vi "Write Timeout.vi"(8 "error in (no error)":errorcluster, 10 "Timeout time(-1ms)":i32=-1, 11 "Interruptible Reply Core in":refnum<class "Interruptible Reply Core.lvclass">) -> (0 "error out":errorcluster, 3 "Interruptible Reply Core out":refnum<class "Interruptible Reply Core.lvclass">)   [LabVIEW 2020, in "Publisher.lvlib" / "Interruptible Reply Core.lvclass"]
doc: "Write the timeout time in ms."
uses:
  Interruptible Reply Core.lvclass
  Interruptible Reply Core.lvclass/Interruptible Reply Core.ctl
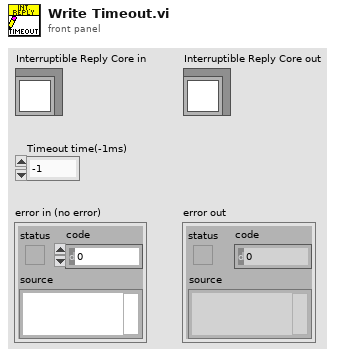
[diagram p1: front panel]
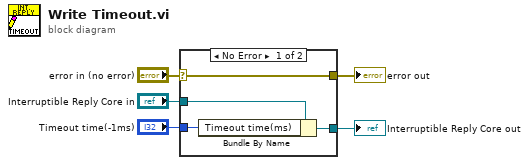
[diagram p0: block diagram]
diagram:
  n1 = case shown="No Error" "error in (no error)" {
    selector: "error in (no error)" -> [w9 w10]
    tunnel: [w9 w10] -> w4
    tunnel: [w7 w11] -> w2
    tunnel: "Interruptible Reply Core in" -> [w8 w11]
    tunnel: "Timeout time(-1ms)" -> [w6 _]
    frame No Error {
      n2 = Bundle By Name(cluster=w8, "Timeout time(ms)"=w6) -> (w7:refnum<class "Interruptible Reply Core.lvclass">)
    }
    frame Error {
    }
  }
  "error out" <- w4
  "Interruptible Reply Core out" <- w2
